vi "Centauro Blinking LED Parser.vi"(8 "error in (no error)":errorcluster, 9 "Read ERD List":T3[](array[typedef])=[{"ERD Number"=61758, "Data Type"=enum."string"}, {"ERD Number"=61755, "Data Type"=enum."string"}, {"ERD Number"=61757, "Data Type"=enum."string"}, {"ERD Number"=61756, "Data Type"=enum."string"}, {"ERD Number"=61751, "Data Type"=enum."string"}] {"ERD Number" format="%.0x"}, 10 "Raw Data In":string) -> (0 "error out":errorcluster, 1 "Blinking LED Binary Number":u32, 2 "LED Status":T2)   [LabVIEW 2016]
uses:
  Common/LabVIEW GEA2 Toolkit/LabVIEW_GEA2_Toolkit.lvlibp/type defs/ERD Read Data In.ctl
  Common/LabVIEW GEA2 Toolkit/LabVIEW_GEA2_Toolkit.lvlibp/type defs/Data Type.ctl
  Centauro Washer/Product Testcode/Centauro/Valew Common/type defs/LED Status OOB.ctl
  Common/LabVIEW GEA2 Toolkit/LabVIEW_GEA2_Toolkit.lvlibp
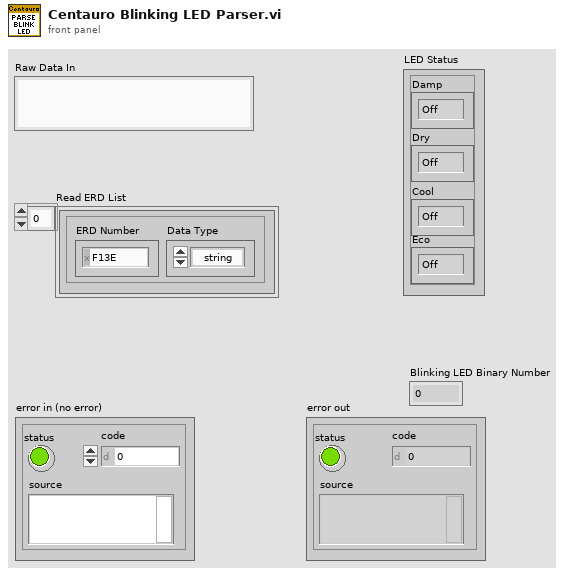
[diagram p1: front panel]
types:
  T1 = typedef "LED Status OOB.ctl" = enum32{"Off", "On", "Blink"}
  T2 = cluster{"Damp":T1, "Dry":T1, "Cool":T1, "Eco":T1}
  T3 = typedef "LabVIEW_GEA2_Toolkit.lvlibp/ERD Read Data In.ctl" = cluster{"ERD Number":u16, "Data Type":T4}
  T4 = typedef "LabVIEW_GEA2_Toolkit.lvlibp/Data Type.ctl" = enum16{"string", "boolean", "uint8_t", "uint16_t", "uint32_t", "uint64_t", "int8_t", "int16_t", "int32_t", "int64_t"}
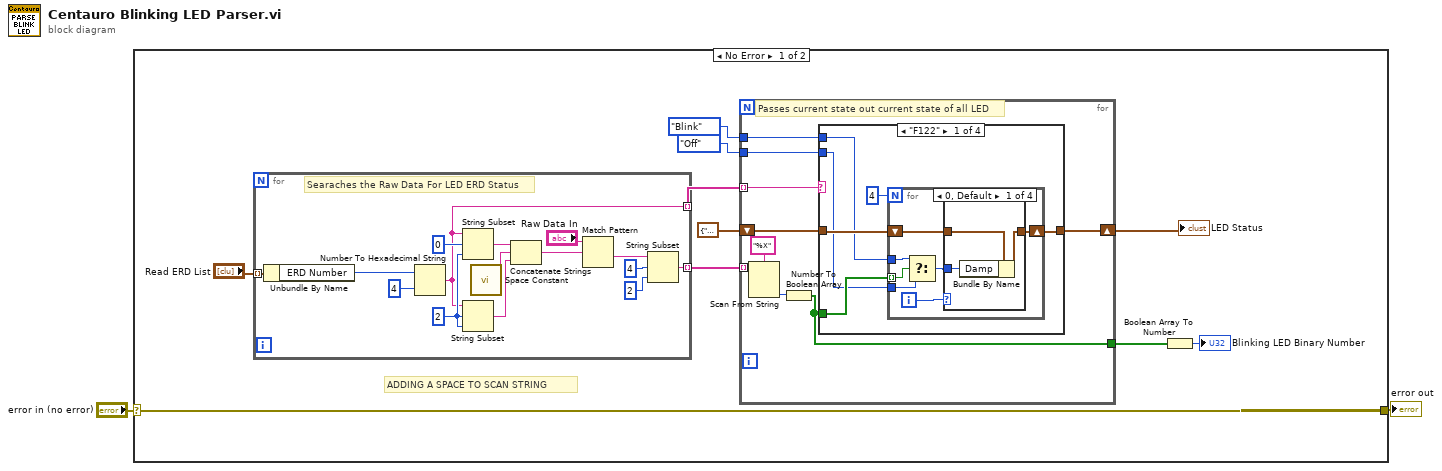
[diagram p0: block diagram]
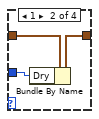
[diagram p2: hidden frame]
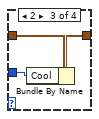
[diagram p3: hidden frame]
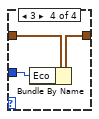
[diagram p4: hidden frame]
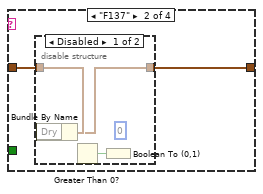
[diagram p5: hidden frame]
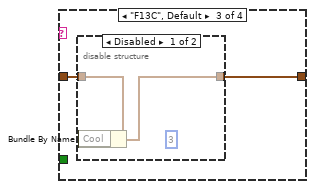
[diagram p7: hidden frame]
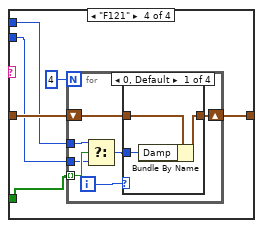
[diagram p9: hidden frame]
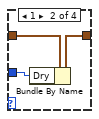
[diagram p10: hidden frame]
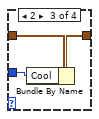
[diagram p11: hidden frame]
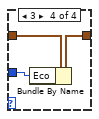
[diagram p12: hidden frame]
diagram:
  n1 = case shown="No Error" "error in (no error)" {
    selector: "error in (no error)" -> [w9 w96]
    tunnel: [w9 w96] -> w1
    frame No Error {
      # "ADDING A SPACE TO SCAN STRING"
      n2 = for {
        tunnel: "Read ERD List" -> [w27] mode=indexing
        tunnel: [w21] -> w11 mode=indexing
        tunnel: [w17] -> w10 mode=indexing
        w19 = 2 ("offset (0)")
        # "Searaches the Raw Data For LED ERD Status"
        n3 = Unbundle By Name(w27) -> ("ERD Number"=w25:u16)
        n4 = Number To Hexadecimal String(1:i16 4 ("width (-)"), 2:w25) -> (0:w17:string)
        n5 = String Subset(string=w17, offset (0)=0 ("length (rest)"), length (rest)=w19) -> (substring=w16:string)
        n6 = String Subset(string=w17, offset (0)=w19, length (rest)=w19) -> (substring=w20:string)
        n7 = call <vilib>:"Space Constant.vi"() -> ("String"=w15:string)
        n8 = Concatenate Strings(w16, w15, w20) -> (w14:string)
        n9 = Match Pattern(string="Raw Data In", regular expression=w14) -> (after substring=w22:string)  [unwired: 1 in, 3 out]
        n10 = String Subset(string=w22, offset (0)=4 ("length (rest)"), length (rest)=2 ("offset (0)")) -> (substring=w21:string)
      }
      n11 = for {
        shift-right: [w35] -> w7
        shift-left: T2 {"Damp"=enum."Off", "Dry"=enum."Off", "Cool"=enum."Off", "Eco"=enum."Off"} ("LED Status") -> [w36]
        tunnel: w11 -> [w33] mode=indexing
        tunnel: w10 -> [w32] mode=indexing
        tunnel: LED_Status_OOB."Off" ("Damp") -> [w31]
        tunnel: LED_Status_OOB."Blink" ("Damp") -> [w30]
        tunnel: [w28] -> w3
        # "Passes current state out current state of all LED"
        n12 = Scan From String(format string="%X", input string=w33) -> (output 1=w29:u32)  [unwired: 3 in, 3 out]
        n13 = Number To Boolean Array(number=w29) -> (Boolean array=w28:bool[])
        n14 = case shown="\"F122\"" w32 {
          tunnel: w36 -> [w41 w63 w68 w76]
          tunnel: [w40 w62 w67 w75] -> w35
          tunnel: w31 -> [w37 _ _ w74]
          tunnel: w30 -> [w38 _ _ w73]
          tunnel: w28 -> [w39 _ _ w72]
          frame "F122" {
            n15 = for {
              N: 4 -> [_]
              shift-right: [w48] -> w40
              shift-left: w41 -> [w49]
              tunnel: w39 -> [w44] mode=indexing
              tunnel: w38 -> [w46]
              tunnel: w37 -> [w43]
              i -> [w47]
              n16 = Select(t=w46, s=w44, f=w43) -> (s? t:f=w45:T1)
              n17 = case shown="0, Default" w47 {
                tunnel: w49 -> [w51 w55 w58 w61]
                tunnel: [w50 w54 w57 w60] -> w48
                tunnel: w45 -> [w52 w53 w56 w59]
                frame 0, Default {
                  n18 = Bundle By Name(cluster=w51, "Damp"=w52) -> (w50:T2)
                }
                frame 1 {
                  n19 = Bundle By Name(cluster=w55, "Dry"=w53) -> (w54:T2)
                }
                frame 2 {
                  n20 = Bundle By Name(cluster=w58, "Cool"=w56) -> (w57:T2)
                }
                frame 3 {
                  n21 = Bundle By Name(cluster=w61, "Eco"=w59) -> (w60:T2)
                }
              }
            }
          }
          frame "F137" {
            n22 = disable-structure shown="Disabled" {
              disable-tunnel: w63 -> [w66 _]
              disable-tunnel: [w65 _] -> w62
              frame Disabled {
                (unwired) 0 ("index")
                n23 = Bundle By Name(cluster=w66) -> (w65:T2)  [unwired: 1 in]
                n24 = Greater Than 0?() -> (x > 0?=w64:bool)  [unwired: 1 in]
                n25 = Boolean To (0,1)(Boolean=w64) -> ()  [unwired: 1 out]
              }
              frame Enabled {
              }
            }
          }
          frame "F13C", Default {
            n26 = disable-structure shown="Disabled" {
              disable-tunnel: w68 -> [w70 _]
              disable-tunnel: [w69 _] -> w67
              frame Disabled {
                (unwired) 3 ("index")
                n27 = Bundle By Name(cluster=w70) -> (w69:T2)  [unwired: 1 in]
              }
              frame Enabled {
              }
            }
          }
          frame "F121" {
            n28 = for {
              N: 4 -> [_]
              shift-right: [w82] -> w75
              shift-left: w76 -> [w83]
              tunnel: w72 -> [w80] mode=indexing
              tunnel: w74 -> [w79]
              tunnel: w73 -> [w78]
              i -> [w81]
              n29 = Select(t=w78, s=w80, f=w79) -> (s? t:f=w77:T1)
              n30 = case shown="0, Default" w81 {
                tunnel: w83 -> [w85 w89 w92 w95]
                tunnel: [w84 w88 w91 w94] -> w82
                tunnel: w77 -> [w86 w87 w90 w93]
                frame 0, Default {
                  n31 = Bundle By Name(cluster=w85, "Damp"=w86) -> (w84:T2)
                }
                frame 1 {
                  n32 = Bundle By Name(cluster=w89, "Dry"=w87) -> (w88:T2)
                }
                frame 2 {
                  n33 = Bundle By Name(cluster=w92, "Cool"=w90) -> (w91:T2)
                }
                frame 3 {
                  n34 = Bundle By Name(cluster=w95, "Eco"=w93) -> (w94:T2)
                }
              }
            }
          }
        }
      }
      "LED Status" <- w7
      n35 = Boolean Array To Number(Boolean array=w3) -> (number=→"Blinking LED Binary Number":u32)
    }
    frame Error {
    }
  }
  "error out" <- w1
